vi "AH_ERRtoSTR.vi"(10 "Error":i32) -> (2 "String Out":string)   [LabVIEW 2021]
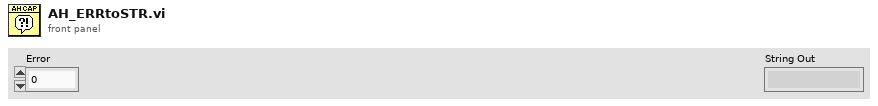
[diagram p1: front panel]
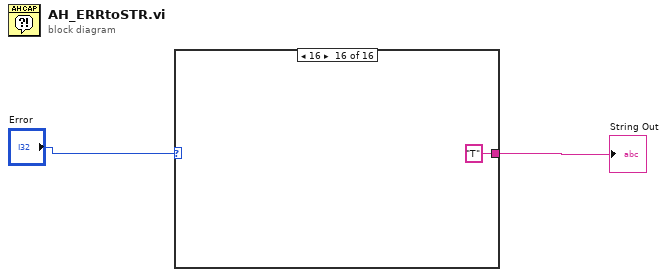
[diagram p0: block diagram]
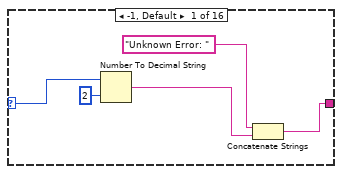
[diagram p2: hidden frame]
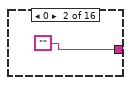
[diagram p3: hidden frame]
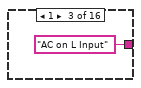
[diagram p4: hidden frame]
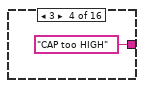
[diagram p5: hidden frame]
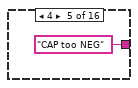
[diagram p6: hidden frame]
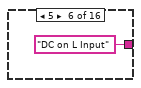
[diagram p7: hidden frame]
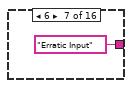
[diagram p8: hidden frame]
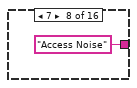
[diagram p9: hidden frame]
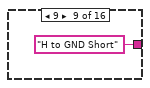
[diagram p10: hidden frame]
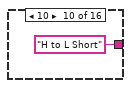
[diagram p11: hidden frame]
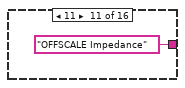
[diagram p12: hidden frame]
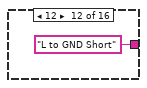
[diagram p13: hidden frame]
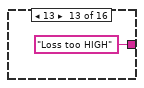
[diagram p14: hidden frame]
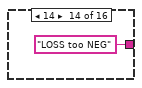
[diagram p15: hidden frame]
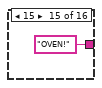
[diagram p16: hidden frame]
diagram:
  n1 = case shown="16" "Error" {
    selector: "Error" -> [w7 _ _ _ _ _ _ _ _ _ _ _ _ _ _ _]
    tunnel: [w3 "" "AC on L Input" "CAP too HIGH" "CAP too NEG" "DC on L Input" "Erratic Input" "Access Noise" "H to GND Short" "H to L Short" "OFFSCALE Impedance" "L to GND Short" "Loss too HIGH" "LOSS too NEG" "OVEN!" "T"] -> w1
    frame -1, Default {
      n2 = Number To Decimal String(number=w7, width (-)=i16 2) -> (decimal integer string=w4:string)
      n3 = Concatenate Strings("Unknown Error: ", w4) -> (w3:string)
    }
    frame 0 {
    }
    frame 1 {
    }
    frame 3 {
    }
    frame 4 {
    }
    frame 5 {
    }
    frame 6 {
    }
    frame 7 {
    }
    frame 9 {
    }
    frame 10 {
    }
    frame 11 {
    }
    frame 12 {
    }
    frame 13 {
    }
    frame 14 {
    }
    frame 15 {
    }
    frame 16 {
    }
  }
  "String Out" <- w1
